vi "Generate Path.vi"() -> (3 "appended path":path)   [LabVIEW 2014, in "Arduino Extra Functions.lvlib"]
uses:
  <vilib>/Aledyne-TSXperts/Arduino Compatible Compiler for LabVIEW/addons/Arduino Extra Functions/Arduino Extra Functions.lvlib
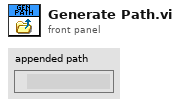
[diagram p1: front panel]
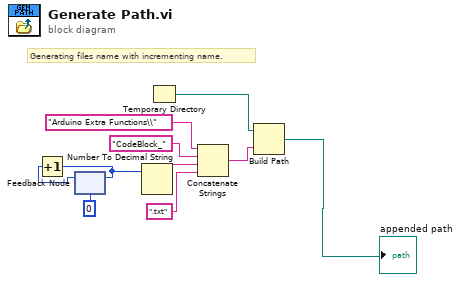
[diagram p0: block diagram]
diagram:
  # "Generating files name with incrementing name."
  n1 = feedback #1(0) -> (w2:i32)
  n2 = Increment(x=w2) -> (x+1=w4:i32)
  n3 = feedback-in #1(w4) -> ()
  n4 = Number To Decimal String(number=w4) -> (decimal integer string=w5:string)  [unwired: 1 in]
  n5 = Temporary Directory() -> (w9:path)
  n6 = Concatenate Strings("Arduino Extra Functions\\" ("string"), "CodeBlock_" ("string"), w5, ".txt" ("string")) -> (w7:string)
  n7 = Build Path(base path=w9, name or relative path=w7) -> (appended path=→"appended path":path)
